vi "EncryptDecryptString.vi"(0 "Original":string, 2 "ROT by...":i32) -> (4 "ROT'd string":string)   [LabVIEW 2022 SP3]
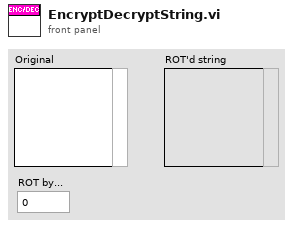
[diagram p1: front panel]
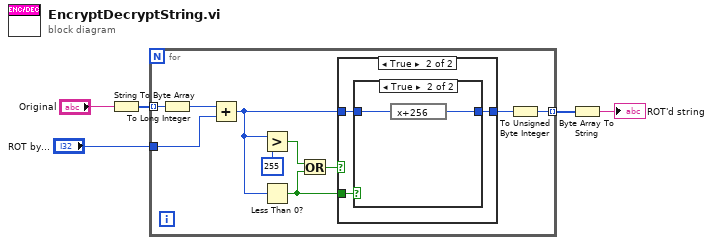
[diagram p0: block diagram]
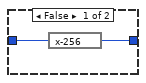
[diagram p3: hidden frame]
diagram:
  n1 = String To Byte Array(string="Original") -> (unsigned byte array=w3:u8[])
  n2 = for {
    tunnel: w3 -> [w15] mode=indexing
    tunnel: [w13] -> w2 mode=indexing
    tunnel: "ROT by..." -> [w12]
    n3 = To Long Integer(number=w15) -> (32bit integer=w14:i32)
    n4 = Add(x=w14, y=w12) -> (x+y=w7:i32)
    n5 = Greater?(x=w7, y=255) -> (0:w8:bool)
    n6 = Less Than 0?(x=w7) -> (x < 0?=w9:bool)
    n7 = Or(x=w8, y=w9) -> (x .or. y?=w10:bool)
    n8 = case shown="True" w10 {
      tunnel: w9 -> [_ w19]
      tunnel: w7 -> [w16 w17]
      tunnel: [w16 w18] -> w6
      frame False {
      }
      frame True {
        n9 = case shown="True" w19 {
          tunnel: [w20 w22] -> w18
          tunnel: w17 -> [w21 w23]
          frame False {
            n10 = expression code="x-256"(w21) -> (w20:i32)
          }
          frame True {
            n11 = expression code="x+256"(w23) -> (w22:i32)
          }
        }
      }
    }
    n12 = To Unsigned Byte Integer(number=w6) -> (unsigned 8bit integer=w13:u8)
  }
  n13 = Byte Array To String(unsigned byte array=w2) -> (string=→"ROT'd string":string)
